vi "Close.vi"(8 "Error In":errorcluster, 11 "Управление ПЛК":T1) -> (0 "error out":errorcluster)   [LabVIEW 2023, in "pump_Lib.lvlib"]
uses:
  pump_Lib.lvlib
  TypeDef/control_Type.ctl
  TypeDef/pump_Type.ctl
  TypeDef/pair_Type.ctl
  TypeDef/parametrs_Type.ctl
panel:
  # "%"
  # "%"
  # "%"
  # "%"
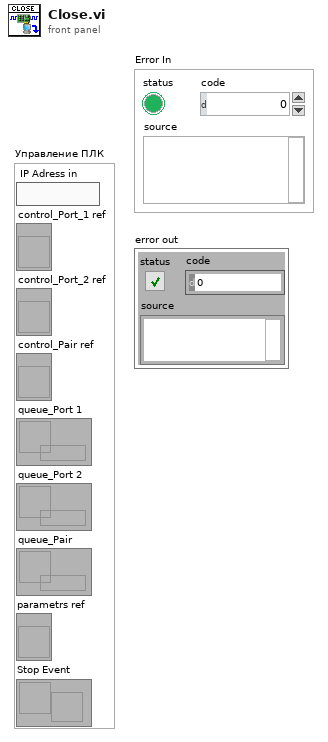
[diagram p1: front panel]
types:
  T1 = typedef "pump_Lib.lvlib/control_Type.ctl" = cluster{"IP Adress in":string, "control_Port_1 ref":refnum<vi>, "control_Port_2 ref":refnum<vi>, "control_Pair ref":refnum<vi>, "queue_Port 1":refnum<queue>, "queue_Port 2":refnum<queue>, "queue_Pair":refnum<queue>, "parametrs ref":refnum<vi>, "Stop Event":refnum<user-event>}
  T2 = typedef "pump_Lib.lvlib/pump_Type.ctl" = cluster{"Давление заданное":dbl, "Давление MAX заданное":dbl, "Давление в насосе":dbl, "Давление в системе":dbl, "Расход заданый":dbl, "Расход текущий":dbl, "Объём заданный":dbl, "Объём текущий":dbl, "Позиция насоса %":dbl, "Ток двигателя":dbl, "controlMsg":string, "Клапан k_sys":bool, "Клапан k_res":bool, "Клапан k_air":bool, "Вверх":bool, "Домой":bool, "Вниз":bool, "Старт расход":bool, "Старт давление":bool, "Сброс объёма":bool, "Сброс давления Рсис":bool, "Сброс давления Рнас":bool, "Bits":cluster{"plc_control":bool, "lag_control":bool, "mstop_control":bool, "st_home":bool, "error":bool, "mstart":bool, "pair":bool, "startQ":bool, "startP":bool, "volume_Stop":bool}}
  T3 = typedef "pump_Lib.lvlib/pair_Type.ctl" = cluster{"Давление заданное":dbl, "Давление в системе":dbl, "Расход заданый":dbl, "Расход текущий":dbl, "Объём заданный":dbl, "Объём текущий":dbl, "Старт давление":bool, "Старт расход":bool, "Сброс объёма":bool, "plc_control":bool, "lag_control":bool, "mstop_control":bool, "Давление":cluster{"АЦП CH 0":dbl, "АЦП CH 1":dbl, "АЦП CH 2":dbl, "АЦП CH 3":dbl, "АЦП CH 4":dbl, "АЦП CH 5":dbl, "АЦП CH 6":dbl, "АЦП CH 7":dbl}, "Modbus":cluster{"Массив чтения":u16[], "Массив записи":u16[]}}
  T4 = enum16{"open", "replace", "create", "open or create", "replace or create", "replace or create with confirmation"}
  T5 = enum16{"big-endian, network order", "native, host order", "little-endian"}
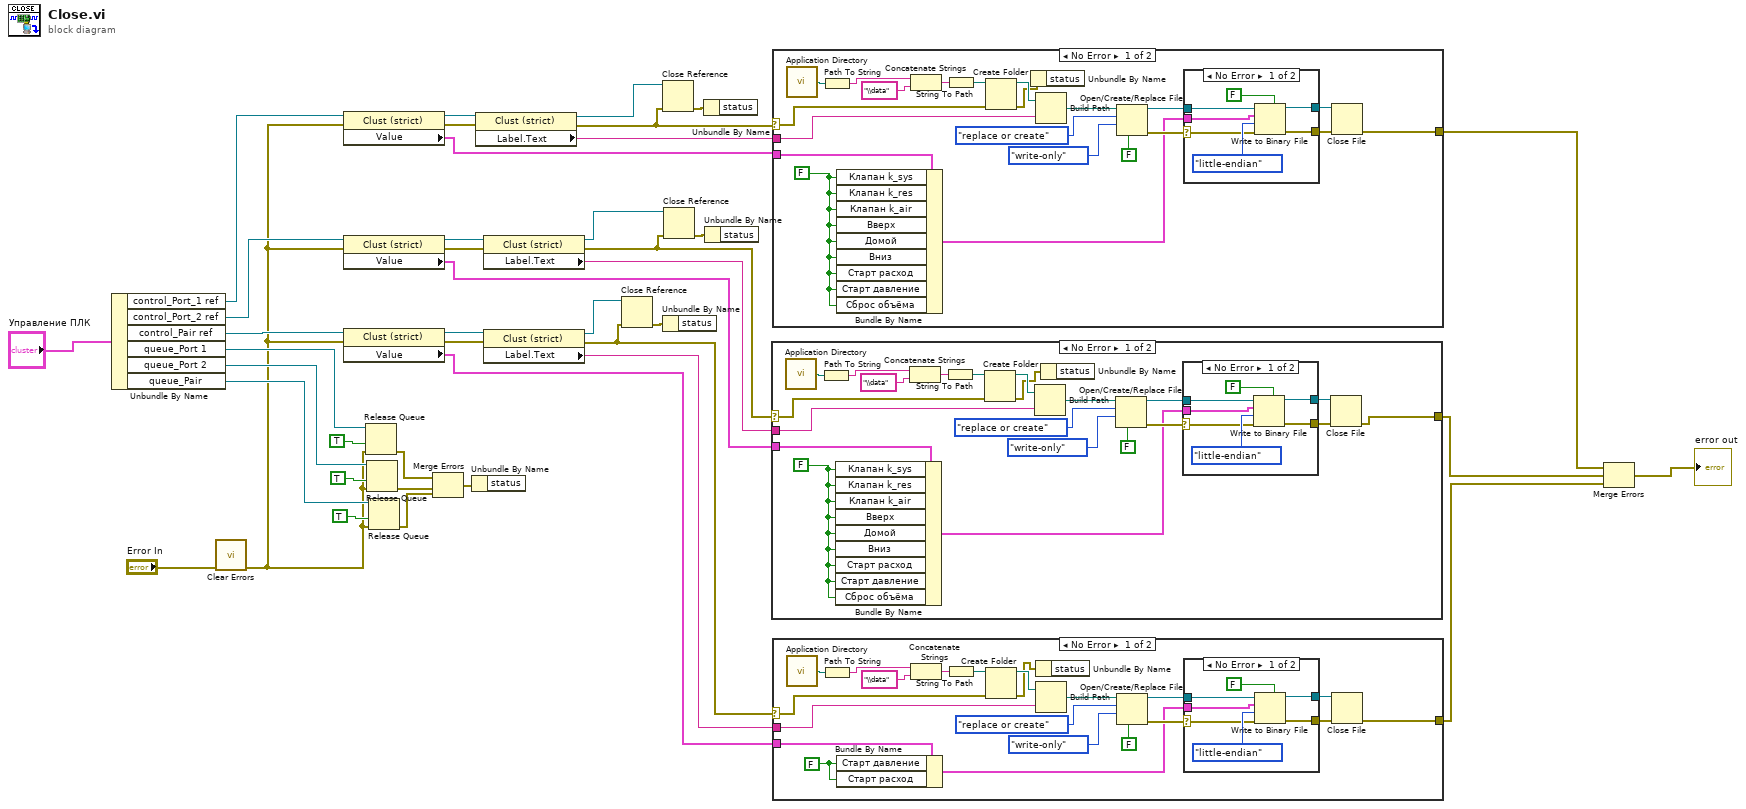
[diagram p0: block diagram]
diagram:
  n1 = Unbundle By Name("Управление ПЛК") -> ("control_Port_1 ref"=w29:refnum<vi>, "control_Port_2 ref"=w28:refnum<vi>, "control_Pair ref"=w27:refnum<vi>, "queue_Port 1"=w37:refnum<queue>, "queue_Port 2"=w36:refnum<queue>, "queue_Pair"=w35:refnum<queue>)
  n2 = call <vilib>:"Clear Errors.vi"("error in (no error)"="Error In") -> ("error out"=w5:errorcluster)  [unwired: 5 in, 1 out]
  n3 = property class="Clust (strict)"(reference=w29, error in=w5) -> (reference out=w26:refnum<vi>, error out=w25:errorcluster, "Value"=w24:T2)
  n4 = property class="Clust (strict)"(reference=w28, error in=w5) -> (reference out=w19:refnum<vi>, error out=w18:errorcluster, "Value"=w15:T2)
  n5 = property class="Clust (strict)"(reference=w27, error in=w5) -> (reference out=w6:refnum<vi>, error out=w7:errorcluster, "Value"=w13:T3)
  n6 = Release Queue(queue=w37, force destroy? (F)=TRUE, error in (no error)=w5) -> (error out=w34:errorcluster)  [unwired: 2 out]
  n7 = Release Queue(queue=w36, force destroy? (F)=TRUE, error in (no error)=w5) -> (error out=w33:errorcluster)  [unwired: 2 out]
  n8 = Release Queue(queue=w35, force destroy? (F)=TRUE, error in (no error)=w5) -> (error out=w32:errorcluster)  [unwired: 2 out]
  n9 = Merge Errors(w34, w33, w32) -> (w31:errorcluster)
  n10 = Unbundle By Name(w31) -> ()  [unwired: 1 out]
  n11 = property class="Clust (strict)"(reference=w26, error in=w25) -> (reference out=w22:refnum<vi>, error out=w21:errorcluster, "Label.Text"=w23:string)
  n12 = property class="Clust (strict)"(reference=w19, error in=w18) -> (reference out=w12:refnum<vi>, error out=w11:errorcluster, "Label.Text"=w16:string)
  n13 = property class="Clust (strict)"(reference=w6, error in=w7) -> (reference out=w10:refnum<vi>, error out=w9:errorcluster, "Label.Text"=w14:string)
  n14 = Close Reference(reference=w10, error in (no error)=w9) -> (error out=w8:errorcluster)
  n15 = Close Reference(reference=w22, error in (no error)=w21) -> (error out=w20:errorcluster)
  n16 = Unbundle By Name(w8) -> ()  [unwired: 1 out]
  n17 = Close Reference(reference=w12, error in (no error)=w11) -> (error out=w17:errorcluster)
  n18 = Unbundle By Name(w20) -> ()  [unwired: 1 out]
  n19 = Unbundle By Name(w17) -> ()  [unwired: 1 out]
  n20 = case shown="No Error" w11 {
    selector: w11 -> [w48 w72]
    tunnel: w15 -> [w46 _]
    tunnel: w16 -> [w47 _]
    tunnel: [w42 w72] -> w2
    frame No Error {
      w45 = FALSE ("K11")
      n21 = call <vilib>:"Application Directory.vi"() -> ("Application Directory"=w60:path)
      n22 = Path To String(path=w60) -> (string=w59:string)
      n23 = Bundle By Name(cluster=w46, "Клапан k_sys"=w45, "Клапан k_res"=w45, "Клапан k_air"=w45, "Вверх"=w45, "Домой"=w45, "Вниз"=w45, "Старт расход"=w45, "Старт давление"=w45, "Сброс объёма"=w45) -> (w44:T2)
      n24 = Concatenate Strings(w59, "\\data" ("string")) -> (w56:string)
      n25 = String To Path(string=w56) -> (path=w55:path)
      n26 = Create Folder(path (use dialog)=w55, error in=w48) -> (created path=w53:path, error out=w43:errorcluster)  [unwired: 1 in, 1 out]
      n27 = Build Path(base path=w53, name or relative path=w47) -> (appended path=w52:path)
      n28 = Unbundle By Name(w43) -> ()  [unwired: 1 out]
      n29 = Open/Create/Replace File(file path (use dialog)=w52, operation (0:open)=T4."replace or create", access (0:read/write)=enum16{"read/write", "read-only", "write-only"}."write-only", disable buffering (F)=FALSE) -> (refnum out=w61:refnum<file>, error out=w62:errorcluster)  [unwired: 2 in, 1 out]
      n30 = case shown="No Error" w62 {
        selector: w62 -> [w67 w71]
        tunnel: w61 -> [w69 w70]
        tunnel: [w66 w71] -> w58
        tunnel: [w65 w70] -> w57
        tunnel: w44 -> [w63 _]
        frame No Error {
          n31 = Write to Binary File(file (use dialog)=w69, data=w63, error in=w67, 5:FALSE ("prepend array or string size? (T)"), 9:T5."little-endian" ("byte order (0:big-endian, network order)")) -> (refnum out=w65:refnum<file>, error out=w66:errorcluster)  [unwired: 1 in, 1 out]
        }
        frame Error {
        }
      }
      n32 = Close File(refnum=w57, error in=w58) -> (error out=w42:errorcluster)  [unwired: 1 out]
    }
    frame Error {
    }
  }
  n33 = case shown="No Error" w21 {
    selector: w21 -> [w79 w103]
    tunnel: w24 -> [w77 _]
    tunnel: w23 -> [w78 _]
    tunnel: [w73 w103] -> w4
    frame No Error {
      w76 = FALSE ("K11")
      n34 = call <vilib>:"Application Directory.vi"() -> ("Application Directory"=w91:path)
      n35 = Path To String(path=w91) -> (string=w90:string)
      n36 = Bundle By Name(cluster=w77, "Клапан k_sys"=w76, "Клапан k_res"=w76, "Клапан k_air"=w76, "Вверх"=w76, "Домой"=w76, "Вниз"=w76, "Старт расход"=w76, "Старт давление"=w76, "Сброс объёма"=w76) -> (w75:T2)
      n37 = Concatenate Strings(w90, "\\data" ("string")) -> (w87:string)
      n38 = String To Path(string=w87) -> (path=w86:path)
      n39 = Create Folder(path (use dialog)=w86, error in=w79) -> (created path=w84:path, error out=w74:errorcluster)  [unwired: 1 in, 1 out]
      n40 = Unbundle By Name(w74) -> ()  [unwired: 1 out]
      n41 = Build Path(base path=w84, name or relative path=w78) -> (appended path=w83:path)
      n42 = Open/Create/Replace File(file path (use dialog)=w83, operation (0:open)=T4."replace or create", access (0:read/write)=enum16{"read/write", "read-only", "write-only"}."write-only", disable buffering (F)=FALSE) -> (refnum out=w92:refnum<file>, error out=w93:errorcluster)  [unwired: 2 in, 1 out]
      n43 = case shown="No Error" w93 {
        selector: w93 -> [w98 w102]
        tunnel: w92 -> [w100 w101]
        tunnel: [w97 w102] -> w89
        tunnel: [w96 w101] -> w88
        tunnel: w75 -> [w94 _]
        frame No Error {
          n44 = Write to Binary File(file (use dialog)=w100, data=w94, error in=w98, 5:FALSE ("prepend array or string size? (T)"), 9:T5."little-endian" ("byte order (0:big-endian, network order)")) -> (refnum out=w96:refnum<file>, error out=w97:errorcluster)  [unwired: 1 in, 1 out]
        }
        frame Error {
        }
      }
      n45 = Close File(refnum=w88, error in=w89) -> (error out=w73:errorcluster)  [unwired: 1 out]
    }
    frame Error {
    }
  }
  n46 = case shown="No Error" w9 {
    selector: w9 -> [w110 w134]
    tunnel: w13 -> [w108 _]
    tunnel: w14 -> [w109 _]
    tunnel: [w104 w134] -> w1
    frame No Error {
      w106 = FALSE ("K11")
      n47 = call <vilib>:"Application Directory.vi"() -> ("Application Directory"=w122:path)
      n48 = Path To String(path=w122) -> (string=w121:string)
      n49 = Bundle By Name(cluster=w108, "Старт давление"=w106, "Старт расход"=w106) -> (w107:T3)
      n50 = Concatenate Strings(w121, "\\data" ("string")) -> (w118:string)
      n51 = String To Path(string=w118) -> (path=w117:path)
      n52 = Create Folder(path (use dialog)=w117, error in=w110) -> (created path=w115:path, error out=w105:errorcluster)  [unwired: 1 in, 1 out]
      n53 = Unbundle By Name(w105) -> ()  [unwired: 1 out]
      n54 = Build Path(base path=w115, name or relative path=w109) -> (appended path=w114:path)
      n55 = Open/Create/Replace File(file path (use dialog)=w114, operation (0:open)=T4."replace or create", access (0:read/write)=enum16{"read/write", "read-only", "write-only"}."write-only", disable buffering (F)=FALSE) -> (refnum out=w123:refnum<file>, error out=w124:errorcluster)  [unwired: 2 in, 1 out]
      n56 = case shown="No Error" w124 {
        selector: w124 -> [w129 w133]
        tunnel: w123 -> [w131 w132]
        tunnel: [w128 w133] -> w120
        tunnel: [w127 w132] -> w119
        tunnel: w107 -> [w125 _]
        frame No Error {
          n57 = Write to Binary File(file (use dialog)=w131, data=w125, error in=w129, 5:FALSE ("prepend array or string size? (T)"), 9:T5."little-endian" ("byte order (0:big-endian, network order)")) -> (refnum out=w127:refnum<file>, error out=w128:errorcluster)  [unwired: 1 in, 1 out]
        }
        frame Error {
        }
      }
      n58 = Close File(refnum=w119, error in=w120) -> (error out=w104:errorcluster)  [unwired: 1 out]
    }
    frame Error {
    }
  }
  n59 = Merge Errors(w4, w2, w1) -> (→"error out":errorcluster)
